vi "New.vi"(6 "Sensor ID (For Sensor Type)":string, 8 "error in (no error)":errorcluster, 9 "Scale Params (Not Sensor)":dbl[](array[numeric]), 10 "Parent":refnum<class "Config Element.lvclass">, 11 "Scale Type":T1) -> (0 "error out":errorcluster, 3 "Scale out":refnum<class "Scale Config.lvclass">)   [LabVIEW 2023, in "VolatusConfig.lvlib" / "Scale Config.lvclass"]
uses:
  Scale Config.lvclass
  lv-cdm/CDM-Config/Config Element/Config Element.lvclass
  Scale Type.ctl
  Meta Type.ctl
  lv-cdm/CDM-Config/Value Type.ctl
  lv-cdm/CDM-Config/Config Element/Write Variant Value.vi
  Scale Config.lvclass/Scale Config.ctl
  VolatusConfigElement/VolatusConfigElement.lvclass
  lv-cdm/CDM-Config/CDM-Config.lvlib
  VolatusConfig.lvlib
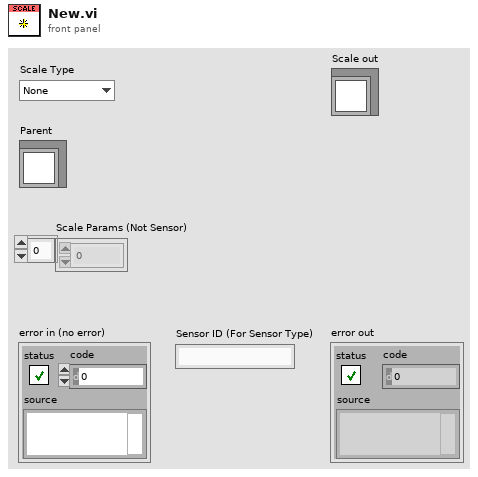
[diagram p1: front panel]
types:
  T1 = typedef "VolatusConfig.lvlib/Scale Type.ctl" = enum16{"None", "Sensor", "Polynomial", "Threshold", "Invert Bool", "Exponential"}
  T2 = typedef "VolatusConfig.lvlib/Meta Type.ctl" = enum16{"UNKNOWN", "VL_System", "VL_Cluster", "VL_Node", "VL_Task", "VL_Group", "VL_Channel", "VL_Task_List", "VL_Scaling", "VL_Sensor", "VL_Sensor_List", "VL_Scale"}
  T3 = typedef "CDM-Config.lvlib/Value Type.ctl" = enum16{"String", "Number", "Bool", "Object", "Array"}
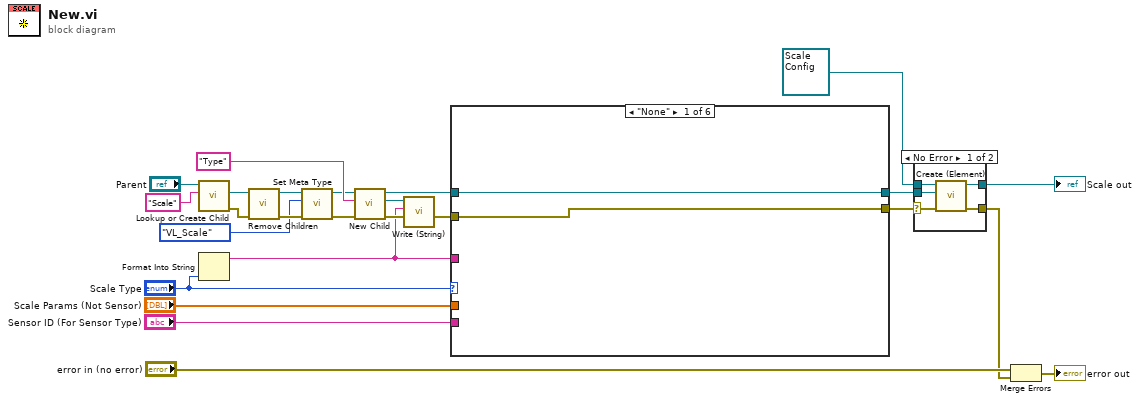
[diagram p0: block diagram]
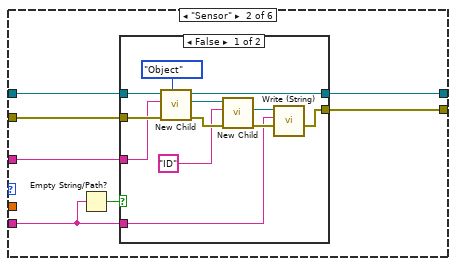
[diagram p2: hidden frame]
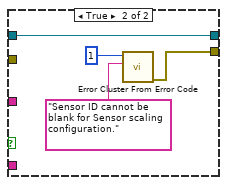
[diagram p3: hidden frame]
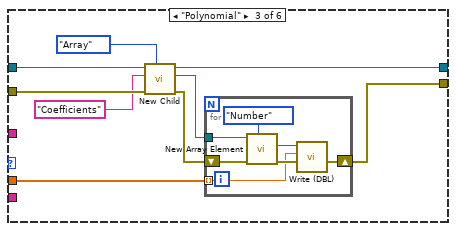
[diagram p4: hidden frame]
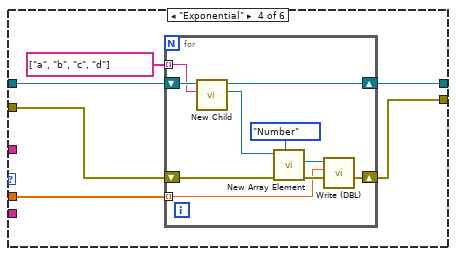
[diagram p5: hidden frame]
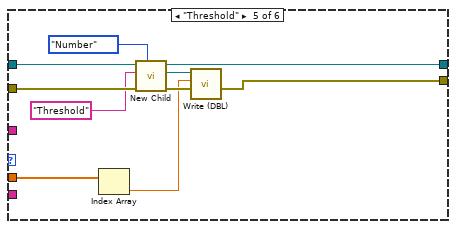
[diagram p6: hidden frame]
diagram:
  n1 = call "Lookup or Create Child.vi"("Name"="Scale" ("Child Name"), "Config Element in"="Parent") -> ("error out"=w6:errorcluster, "Child"=w7:refnum<class "Config Element.lvclass">)  [unwired: 6 in, 2 out]
  n2 = Format Into String("Scale Type") -> (resulting string=w11:string)  [unwired: 3 in, 1 out]
  n3 = call "Remove Children.vi"("error in (no error)"=w6, "Config Element in"=w7) -> ("error out"=w5:errorcluster, "Config Element out"=w3:refnum<class "Config Element.lvclass">)  [unwired: 8 in]
  n4 = call "Set Meta Type.vi"("error in (no error)"=w5, "Meta Type"=Meta_Type."VL_Scale", "Element In"=w3) -> ("error out"=w4:errorcluster, "Element"=w2:refnum<class "Config Element.lvclass">)  [unwired: 7 in]
  n5 = call "New Child.vi"("error in (no error)"=w4, "Child Name"="Type", "Config Element in"=w2) -> ("error out"=w25:errorcluster, "New Child"=w19:refnum<class "Config Element.lvclass">, "Config Element out"=w18:refnum<class "Config Element.lvclass">)  [unwired: 6 in]
  n6 = call "Write (String).vi"("error in (no error)"=w25, "String Value"=w11, "Config Element in"=w19) -> ("error out"=w17:errorcluster)  [unwired: 7 in, 1 out]
  n7 = case shown="\"None\"" "Scale Type" {
    tunnel: w18 -> [w27 w33 w58 w70 w91 w92]
    tunnel: w17 -> [w26 w34 w57 w66 w90 w93]
    tunnel: "Scale Params (Not Sensor)" -> [_ _ w54 w68 w85 _]
    tunnel: "Sensor ID (For Sensor Type)" -> [_ w29 _ _ _ _]
    tunnel: [w27 w31 w51 w67 w82 w92] -> w12
    tunnel: w11 -> [_ w32 _ _ _ _]
    tunnel: [w26 w30 w52 w71 w83 w93] -> w10
    frame "None" {
    }
    frame "Sensor" {
      n8 = Empty String/Path?(string/path=w29) -> (empty?=w28:bool)
      n9 = case shown="False" w28 {
        tunnel: w34 -> [w45 _]
        tunnel: w33 -> [w44 w50]
        tunnel: w32 -> [w43 _]
        tunnel: [w37 w50] -> w31
        tunnel: [w36 w49] -> w30
        tunnel: w29 -> [w35 _]
        frame False {
          n10 = call "New Child.vi"("Value Type (Object)"=Value_Type."Object" ("Value Type (String)"), "error in (no error)"=w45, "Child Name"=w43, "Config Element in"=w44) -> ("error out"=w46:errorcluster, "New Child"=w41:refnum<class "Config Element.lvclass">, "Config Element out"=w37:refnum<class "Config Element.lvclass">)  [unwired: 5 in]
          n11 = call "New Child.vi"("error in (no error)"=w46, "Child Name"="ID", "Config Element in"=w41) -> ("error out"=w39:errorcluster, "New Child"=w38:refnum<class "Config Element.lvclass">)  [unwired: 6 in, 1 out]
          n12 = call "Write (String).vi"("error in (no error)"=w39, "String Value"=w35, "Config Element in"=w38) -> ("error out"=w36:errorcluster)  [unwired: 7 in, 1 out]
        }
        frame True {
          n13 = call <vilib>:"Error Cluster From Error Code.vi"("error message (\"\")"="Sensor ID cannot be blank for Sensor scaling configuration.", "error code (0)"=1) -> ("error out"=w49:errorcluster)  [unwired: 7 in]
        }
      }
    }
    frame "Polynomial" {
      n14 = call "New Child.vi"("Value Type (Object)"=Value_Type."Array" ("Value Type (String)"), "error in (no error)"=w57, "Child Name"="Coefficients", "Config Element in"=w58) -> ("error out"=w53:errorcluster, "New Child"=w51:refnum<class "Config Element.lvclass">)  [unwired: 5 in, 1 out]
      n15 = for {
        tunnel: w54 -> [w60] mode=indexing
        tunnel: w51 -> [w65]
        shift-right: [w59] -> w52
        shift-left: w53 -> [w63]
        n16 = call "New Array Element.vi"("Value Type (String)"=Value_Type."Number", "error in (no error)"=w63, "Config Element in"=w65) -> ("error out"=w62:errorcluster, "New Child"=w61:refnum<class "Config Element.lvclass">)  [unwired: 5 in, 2 out]
        n17 = call "Write (DBL).vi"("error in (no error)"=w62, "DBL Value"=w60, "Config Element in"=w61) -> ("error out"=w59:errorcluster)  [unwired: 7 in, 1 out]
      }
    }
    frame "Exponential" {
      n18 = for {
        tunnel: w68 -> [w77] mode=indexing
        shift-right: [w76] -> w71
        shift-left: w66 -> [w80]
        shift-right: [w74] -> w67
        shift-left: w70 -> [w75]
        tunnel: string[] ["a", "b", "c", "d"] -> [w73] mode=indexing
        n19 = call "New Child.vi"("Child Name"=w73, "Config Element in"=w75) -> ("New Child"=w72:refnum<class "Config Element.lvclass">, "Config Element out"=w74:refnum<class "Config Element.lvclass">)  [unwired: 7 in, 1 out]
        n20 = call "New Array Element.vi"("Value Type (String)"=Value_Type."Number", "error in (no error)"=w80, "Config Element in"=w72) -> ("error out"=w79:errorcluster, "New Child"=w78:refnum<class "Config Element.lvclass">)  [unwired: 5 in, 2 out]
        n21 = call "Write (DBL).vi"("error in (no error)"=w79, "DBL Value"=w77, "Config Element in"=w78) -> ("error out"=w76:errorcluster)  [unwired: 7 in, 1 out]
      }
    }
    frame "Threshold" {
      n22 = Index Array(array=w85) -> (element=w84:dbl)  [unwired: 1 in]
      n23 = call "New Child.vi"("Value Type (Object)"=Value_Type."Number" ("Value Type (String)"), "error in (no error)"=w90, "Child Name"="Threshold", "Config Element in"=w91) -> ("error out"=w87:errorcluster, "New Child"=w86:refnum<class "Config Element.lvclass">, "Config Element out"=w82:refnum<class "Config Element.lvclass">)  [unwired: 5 in]
      n24 = call "Write (DBL).vi"("error in (no error)"=w87, "DBL Value"=w84, "Config Element in"=w86) -> ("error out"=w83:errorcluster)  [unwired: 7 in, 1 out]
    }
    frame "Invert Bool" {
    }
  }
  n25 = case shown="No Error" w10 {
    selector: w10 -> [w95 w99]
    tunnel: refnum<class "Scale Config.lvclass"> refnum ("Scale in") -> [w98 _]
    tunnel: [w97 _] -> w13
    tunnel: w12 -> [w96 _]
    tunnel: [w94 w99] -> w8
    frame No Error {
      n26 = call "Create (Element).vi"("error in (no error)"=w95, "Element"=w96, "VolatusConfigElement in"=w98) -> ("error out"=w94:errorcluster, "VolatusConfigElement out"=w97:refnum<class "Scale Config.lvclass">)  [unwired: 7 in]
    }
    frame Error {
    }
  }
  "Scale out" <- w13
  n27 = Merge Errors("error in (no error)", w8) -> (→"error out":errorcluster)
